vi "GetCellStrColor.vi"(7 "Color":u32, 8 "error in (no error)":errorcluster, 10 "Hdr Name":T1, 11 "Current in":refnum<class "Current.lvclass">) -> (0 "error out":errorcluster, 1 "Cell String":string, 2 "Cell Color":u32, 3 "Current out":refnum<class "Current.lvclass">)   [LabVIEW 2018, in "Measurement Channels.lvlib" / "Current.lvclass"]
uses:
  Current.lvclass
  Common/Controls/HeaderNames.ctl
  SubVIs Table/Custom Ctls Table/ge_ColType.ctl
  Current.lvclass/Current.ctl
  Class Channel/Channel.lvclass
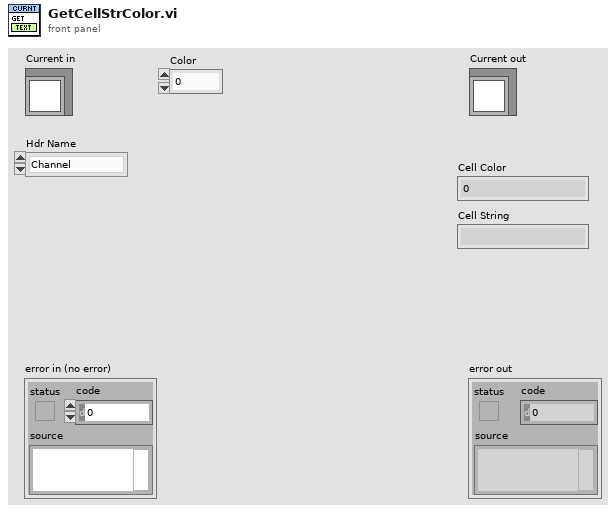
[diagram p1: front panel]
types:
  T1 = typedef "HeaderNames.ctl" = enum16{"Channel", "Device", "Spacer", "Description", "MB", "Range", "Terminal", "Coupling", "Thresh (V)", "Pulse/Rev", "Slope", "Min EU", "Min RPM", "mV/EU", "Iex", "Temp Units", "Type", "CJC Src", "CJC Val", "Ro", "Wire Cfg", "Strain Mode", "Vex", "Bridge Type", "GF", "Gauge Res", "Poisson", "Lead Res", "Init Strain", "GAF", "Scale", "Offset", "Unit (EU)", "dB?", "dB Ref", "Cal Mag", "Cal Units", "Max Temp", "Min Temp", "Max Strain", "Min Strain"}
  T2 = typedef "ge_ColType.ctl" = enum16{"Volts", "Amps", "Ohms", "TermCfg", "WireCfg", "Coup", "Slope", "Iex", "CalUnits", "ThrmUnits", "ThrmType", "CJCSrc", "BrdgType", "Strn Mode", "RTDType"}
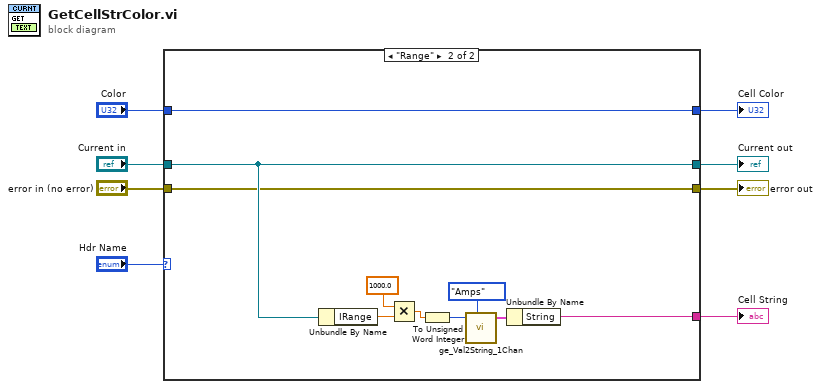
[diagram p0: block diagram]
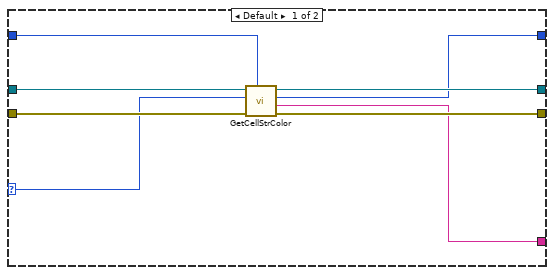
[diagram p2: hidden frame]
diagram:
  n1 = case shown="\"Range\"" "Hdr Name" {
    selector: "Hdr Name" -> [w9 _]
    tunnel: "Current in" -> [w13 w18]
    tunnel: [w10 w20] -> w1
    tunnel: [w14 w19] -> w7
    tunnel: "Color" -> [w15 w19]
    tunnel: [w16 w18] -> w6
    tunnel: "error in (no error)" -> [w12 w17]
    tunnel: [w11 w17] -> w3
    frame Default {
      n2 = call-parent "GetCellStrColor.vi"("Color"=w15, "error in (no error)"=w12, "Hdr Name"=w9, "Channel in"=w13) -> ("error out"=w11:errorcluster, "Cell String"=w10:string, "Cell Color"=w14:u32, "Channel out"=w16:refnum<class "Current.lvclass">)  [unwired: 4 in]
    }
    frame "Range" {
      n3 = Unbundle By Name(w18) -> ("IRange"=w24:dbl)
      n4 = Multiply(x=1000.0, y=w24) -> (x*y=w26:dbl)
      n5 = To Unsigned Word Integer(number=w26) -> (unsigned 16bit integer=w22:u16)
      n6 = call "ge_Val2String_1Chan.vi"("Value"=w22, "ColType"=ge_ColType."Amps") -> ("String and Val"=w21:cluster{"String":string, "Value":u16})  [unwired: 5 in]
      n7 = Unbundle By Name(w21) -> ("String"=w20:string)
    }
  }
  "error out" <- w3
  "Current out" <- w6
  "Cell String" <- w1
  "Cell Color" <- w7
